vi "SetVertical.vi"(8 "error in (no error)":errorcluster, 11 "TektronixDPO in":refnum<class "TektronixDPO_PhysicalDevice.lvclass">) -> (0 "error out":errorcluster, 3 "TektronixDPO_PhysicalDevice.lvclass":refnum<class "TektronixDPO_PhysicalDevice.lvclass">)   [LabVIEW 2013, in "TektronixDPO_PhysicalDevice.lvclass"]
doc: "Send the channel settings to the physical device"
uses:
  TektronixDPO_PhysicalDevice.lvclass
  TektronixDPO_PhysicalDevice.lvclass/TektronixDPO_PhysicalDevice.ctl
  Tektronix DPO MSO 2000 4000 Series/Tektronix DPO MSO 2000 4000 Series.lvlib
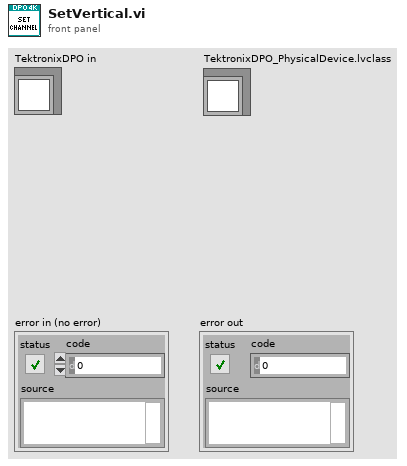
[diagram p1: front panel]
types:
  T1 = typedef "Choice78.ctl" = enum16{"1M", "75", "50"}
  T2 = typedef "Choice80.ctl" = u16
  T3 = typedef "Choice11.ctl" = enum16{"AC", "DC", "Ground"}
  T4 = typedef "Choice79.ctl" = enum16{"FULL", "250 MHz", "150 MHz", "20 MHz"}
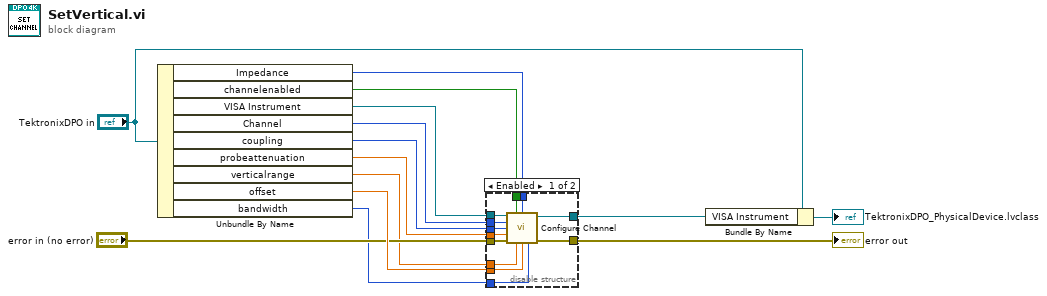
[diagram p0: block diagram]
diagram:
  n1 = Unbundle By Name("TektronixDPO in") -> ("Impedance"=w10:T1, "channelenabled"=w9:bool, "VISA Instrument"=w4:refnum<visa-resource-name>, "Channel"=w3:T2, "coupling"=w7:T3, "probeattenuation"=w8:dbl, "verticalrange"=w6:dbl, "offset"=w14:dbl, "bandwidth"=w5:T4)
  n2 = disable-structure shown="Enabled" {
    disable-tunnel: w14 -> [w26 _]
    disable-tunnel: "error in (no error)" -> [w25 w27]
    disable-tunnel: w10 -> [w24 _]
    disable-tunnel: w9 -> [w23 _]
    disable-tunnel: w8 -> [w22 _]
    disable-tunnel: w7 -> [w21 _]
    disable-tunnel: w6 -> [w20 _]
    disable-tunnel: w5 -> [w19 _]
    disable-tunnel: w4 -> [w18 w28]
    disable-tunnel: w3 -> [w17 _]
    disable-tunnel: [w16 w27] -> w1
    disable-tunnel: [w15 w28] -> w2
    frame Enabled {
      n3 = call "Configure Channel.vi"("VISA resource name"=w18, "Enable Channel (T: Enable)"=w23, "Input Impedance (0: 1M ohm)"=w24, "Channel (0: Channel 1)"=w17, "Vertical Coupling (1: DC)"=w21, "Probe Attenuation (1)"=w22, "error in (no error)"=w25, "Vertical Range (10.0 V)"=w20, "Vertical Offset (0.0 V)"=w26, "Bandwidth (0: FULL)"=w19) -> ("VISA resource name out"=w15:refnum<visa-resource-name>, "error out"=w16:errorcluster)  [unwired: 4 in]
    }
    frame Disabled {
    }
  }
  "error out" <- w1
  n4 = Bundle By Name(cluster="TektronixDPO in", "VISA Instrument"=w2) -> (→"TektronixDPO_PhysicalDevice.lvclass":refnum<class "TektronixDPO_PhysicalDevice.lvclass">)
